vi "Save PNG Image of Front Panel.vi"(8 "error in (no error)":errorcluster, 10 "VI Path":path, 11 "File Path In":path) -> (0 "error out":errorcluster, 3 "File Path Out":path)   [LabVIEW 2022 SP3]
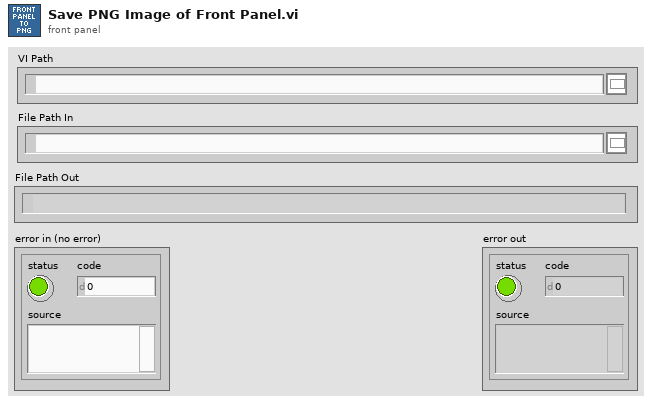
[diagram p1: front panel]
types:
  T1 = typedef "imagedata.ctl" = cluster{"image type":i32, "image depth":i32, "image":u8[], "mask":u8[], "colors":u32[], "Rectangle":cluster{"left":i16, "top":i16, "right":i16, "bottom":i16}}
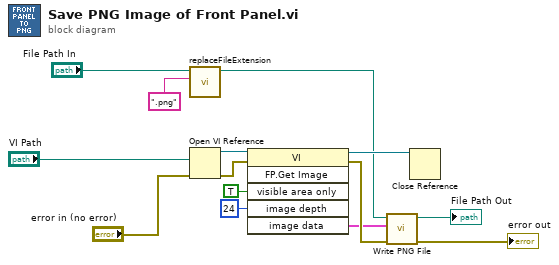
[diagram p0: block diagram]
diagram:
  n1 = call "replaceFileExtension.vi"("replacementExtension"=".png" ("string"), "pathIn"="File Path In") -> ("pathOut"=w3:path)  [unwired: 8 in, 1 out]
  n2 = Open VI Reference(vi path="VI Path", error in (no error)="error in (no error)") -> (vi reference=w7:refnum<vi>, error out=w11:errorcluster)  [unwired: 4 in]
  n3 = invoke class="VI" method="FP.Get Image"(reference=w7, error in=w11, "visible area only"=TRUE ("Visible Area Only"), "image depth"=24 ("Image Depth")) -> (reference out=w6:refnum<vi>, error out=w12:errorcluster, "image data"=w8:T1)  [unwired: 2 in, 3 out]
  n4 = call <vilib>:"Write PNG File.vi"("error in (no error)"=w12, "image data"=w8, "path to PNG file"=w3) -> ("error out"=→"error out":errorcluster, "path"=→"File Path Out":path)  [unwired: 7 in]
  n5 = Close Reference(reference=w6) -> ()  [unwired: 1 in, 1 out]
